vi "callback_send_queue_obtain.vi"(8 "error in (no error)":errorcluster) -> (0 "error out":errorcluster, 3 "queue out":refnum<queue>)   [LabVIEW 2013, in "libssh2_integration_tests.lvlib"]
uses:
  libssh2_integration_tests.lvlib
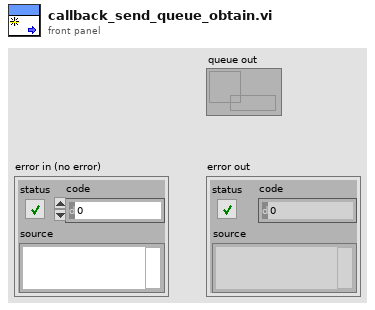
[diagram p1: front panel]
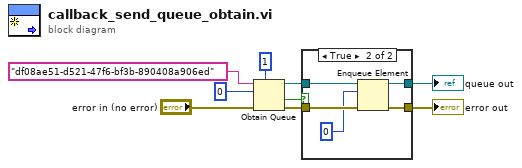
[diagram p0: block diagram]
diagram:
  n1 = Obtain Queue(max queue size (-1, unlimited)=1, name (unnamed)="df08ae51-d521-47f6-bf3b-890408a906ed", element data type=i64 0, error in (no error)="error in (no error)") -> (queue out=w7:refnum<queue>, created new?=w6:bool, error out=w9:errorcluster)  [unwired: 1 in]
  n2 = case shown="True" w6 {
    tunnel: w9 -> [w10 w16]
    tunnel: [w10 w15] -> w3
    tunnel: w7 -> [w11 w14]
    tunnel: [w11 w13] -> w1
    frame False {
    }
    frame True {
      n3 = Enqueue Element(queue=w14, element=0, error in (no error)=w16) -> (queue out=w13:refnum<queue>, error out=w15:errorcluster)  [unwired: 1 in, 1 out]
    }
  }
  "error out" <- w3
  "queue out" <- w1
